vi "ARC_Queue Status.vi"(8 "error in (no error)":errorcluster caption="Error In (no error)", 10 "Return Elements?(F)":bool, 11 "Queue Name":string) -> (0 "error out":errorcluster caption="Error Out", 3 "Queue Status":T1)   [LabVIEW 2016]
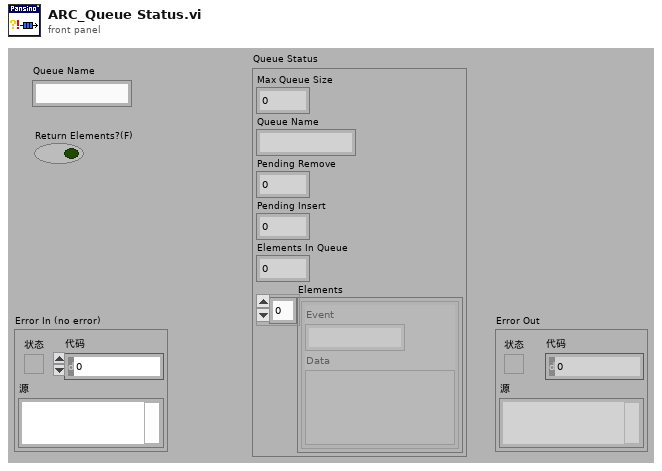
[diagram p1: front panel]
types:
  T1 = cluster{"Max Queue Size":i32, "Queue Name":string, "Pending Remove":i32, "Pending Insert":i32, "Elements In Queue":i32, "Elements":cluster{"Event":string, "Data":variant}[]}
  T2 = cluster{"max queue size":i32, string, "# pending remove":i32, "# pending insert":i32, "# elements in queue":i32, "elements":cluster{"Event":string, "Data":variant}[]}
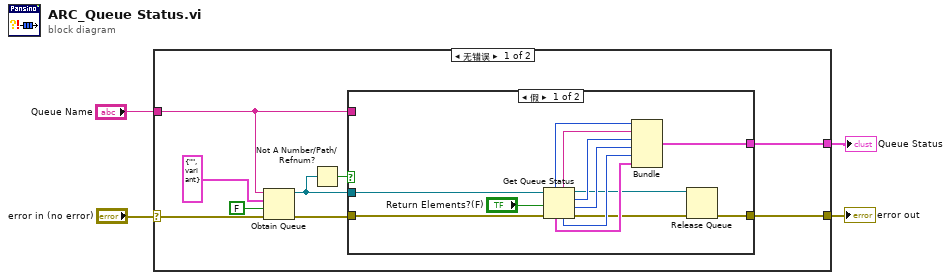
[diagram p0: block diagram]
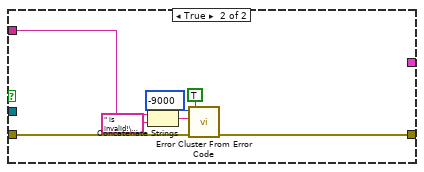
[diagram p2: hidden frame]
diagram:
  n1 = case shown="无错误" "error in (no error)" {
    selector: "error in (no error)" -> [w12 w34]
    tunnel: [w13 w34] -> w3
    tunnel: "Queue Name" -> [w7 _]
    tunnel: [w5 _] -> w1
    frame No Error {
      n2 = Obtain Queue(name (unnamed)=w7, element data type=cluster{"Event":string, "Data":variant} {"Event"="", "Data"=variant} ("输出簇"), create if not found? (T)=FALSE ("如未找到是否创建？(T)"), error in (no error)=w12) -> (queue out=w9:refnum<queue>, error out=w11:errorcluster)  [unwired: 1 in, 1 out]
      n3 = Not A Number/Path/Refnum?(number/path/refnum=w9) -> (NaN/Path/Refnum?=w8:bool)
      n4 = case shown="假" w8 {
        tunnel: w11 -> [w26 w29]
        tunnel: [w19 _] -> w5
        tunnel: [w15 w28] -> w13
        tunnel: w7 -> [_ w27]
        tunnel: w9 -> [w17 _]
        frame False {
          n5 = Get Queue Status(queue=w17, return elements? (F)="Return Elements?(F)", error in (no error)=w26) -> (queue out=w14:refnum<queue>, queue name=w24:string, max queue size=w25:i32, # pending remove=w23:i32, # pending insert=w22:i32, error out=w16:errorcluster, # elements in queue=w21:i32, elements=w20:cluster{"Event":string, "Data":variant}[])
          n6 = Bundle("max queue size"=w25, w24, "# pending remove"=w23, "# pending insert"=w22, "# elements in queue"=w21, "elements"=w20) -> (w19:T2)  [unwired: 1 in]
          n7 = Release Queue(queue=w14, error in (no error)=w16) -> (error out=w15:errorcluster)  [unwired: 1 in, 2 out]
        }
        frame True {
          n8 = Concatenate Strings(w27, " is invalid!\nEnsure the queue has been created!" ("字符串")) -> (w32:string)
          n9 = call <vilib>:"Error Cluster From Error Code.vi"("show call chain? (False)"=TRUE, "error in (no error)"=w29, "error message (\"\")"=w32, "error code (0)"=-9000) -> ("error out"=w28:errorcluster)  [unwired: 5 in]
        }
      }
    }
    frame Error {
    }
  }
  "error out" <- w3
  "Queue Status" <- w1
